vi "init Screen.vi"(8 "error in":errorcluster) -> (0 "error out":errorcluster)   [LabVIEW 2020, in "SimpleDependencyInspector.lvlib"]
uses:
  SimpleDependencyInspector.lvlib
  Image Type--enum.ctl
  Files Selection--cluster.ctl
  File Explorer/File Explorer.lvlib
  <vilib>/Platform/browser.llb/Open URL in Default Browser (string).vi
panel:
  in  "Install Graphviz":bool
  in  "Refresh":bool
  in  "4. Dependency Inspector Working Path":path
  in  "5. Output Image Path":T1
  in  "PPLR":bool caption="Packed Library (*.lvlibp)"
  in  "PPL F":bool caption="Packed Library (*.lvlibp)"
  in  "Virtual Instruments (*.vi) R":bool caption="Virtual Instruments (*.vi)"
  in  "Typedefs(*.ctl) R":bool caption="Typedefs(*.ctl)"
  in  "Class(*.lvclass) R":bool caption="Class(*.lvclass)"
  in  "Libraries(*.lvlib) R":bool caption="Libraries(*.lvlib)"
  in  "Virtual Instruments (*.vi) F":bool caption="Virtual Instruments (*.vi)"
  in  "2. Folder Structure":string[](tree)
  in  "1. LabVIEW Code Folder Container":path
  in  "Typedefs(*.ctl) F":bool caption="Typedefs(*.ctl)"
  in  "Class(*.lvclass) F":bool caption="Class(*.lvclass)"
  in  "Libraries(*.lvlib) F":bool caption="Libraries(*.lvlib)"
  in  "Scan Project":bool caption="8. Find Dependencies from Selection"
  in  "7. Include LV dependencies (vi.lib, usr.lib, etc.)":bool
  # "Instructions:\n1. Choose the folder containing your LabVIEW code.\n2. Select the specific files or folders you want to analyze for dependencies. Use the Shift key to select multiple items.\n3. If you selected folders, specify the LabVIEW file types to include in the analysis.\n4.Specify the Working Path, where the .dot file and dependency image will be saved.\n5. Select the Image type for the dependencies. SVG is the preferred option, LabVIEW cannot handle these images directly. If you choose SVG, the image will be opened in your default browser.\n6.Select the dependency file Types you want to include in your plot.\n7. Decide whether to include all LabVIEW dependencies in the plot. Note that this may result in a large and complex diagram that can be difficult to interpret.\n8.Click the \"Find Dependencies from Selection\" button to begin the analysis."
  # "6. Dependencies to Include in the plot:"
  # "3. Files to Scan for Dependencies in folders:"
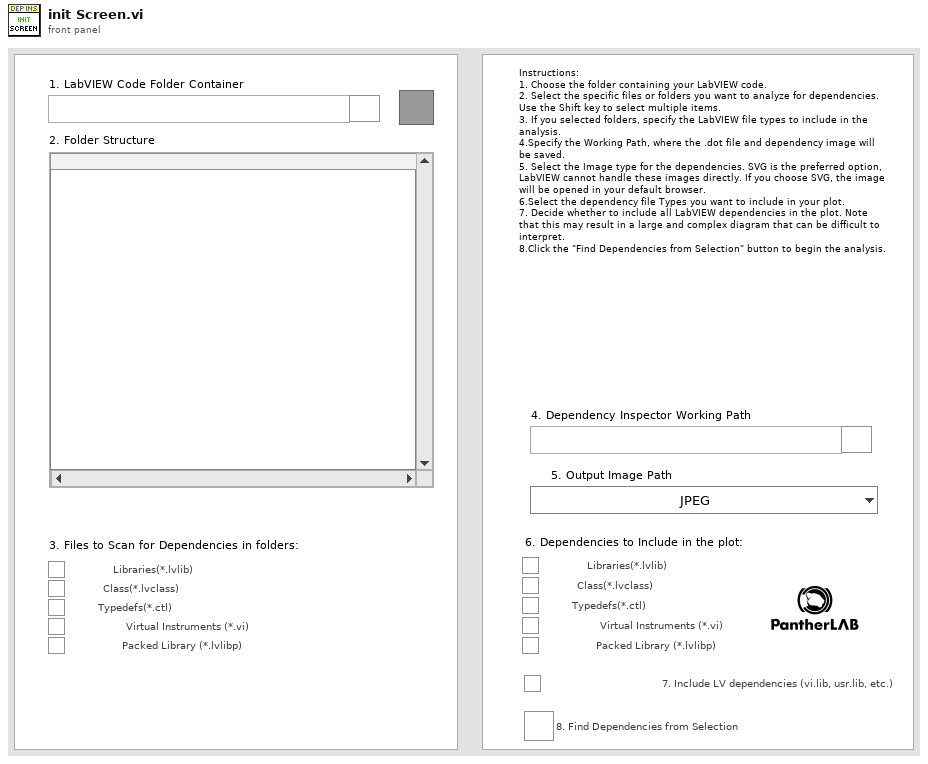
[diagram p1: front panel]
types:
  T1 = typedef "SimpleDependencyInspector.lvlib/Image Type--enum.ctl" = enum16{"JPEG", "PNG", "BMP", "SVG"}
  T2 = typedef "SimpleDependencyInspector.lvlib/Broadcast Events--cluster.ctl" = cluster{"Module Did Init":refnum<user-event>, "Status Updated":refnum<user-event>, "Error Reported":refnum<user-event>, "Module Did Stop":refnum<user-event>, "Update Module Execution Status":refnum<user-event>}
  T3 = typedef "SimpleDependencyInspector.lvlib/Files Selection--cluster.ctl" = cluster{"LVLib":bool, "LVClass":bool, "Typedefs":bool, "vis":bool, "ppl":bool}
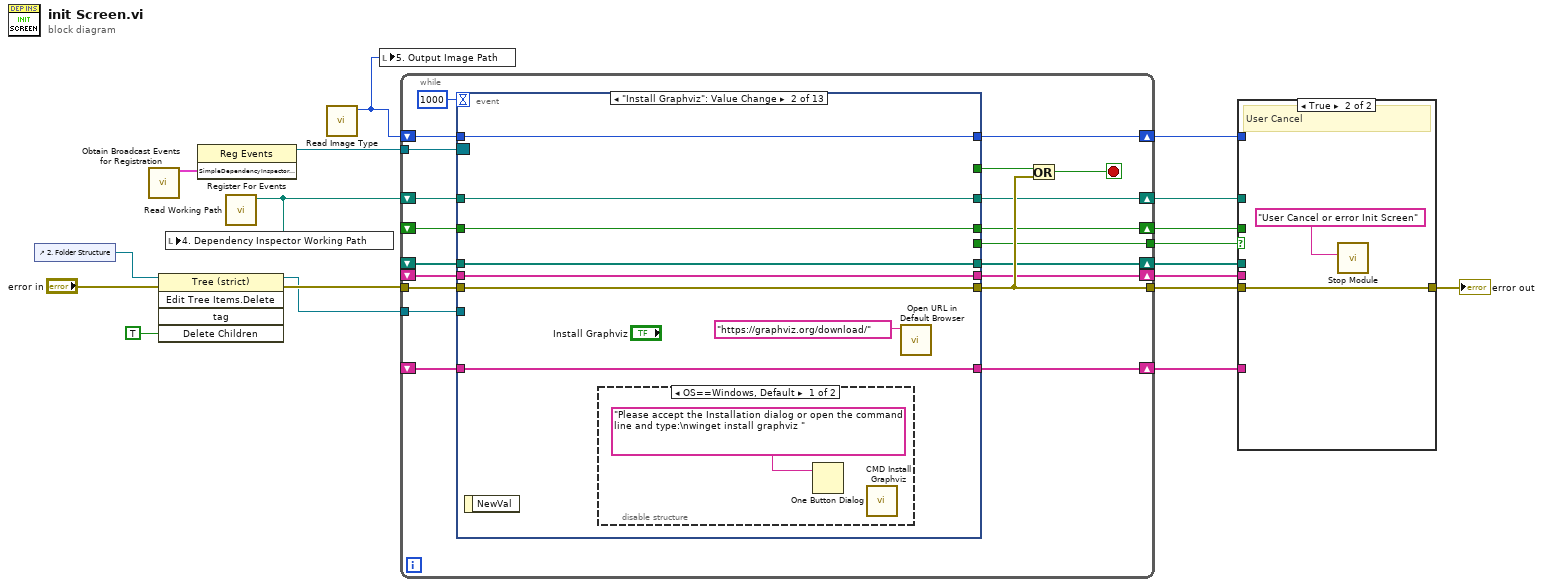
[diagram p0: block diagram]
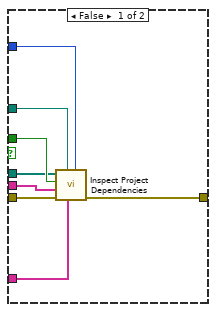
[diagram p2: hidden frame]
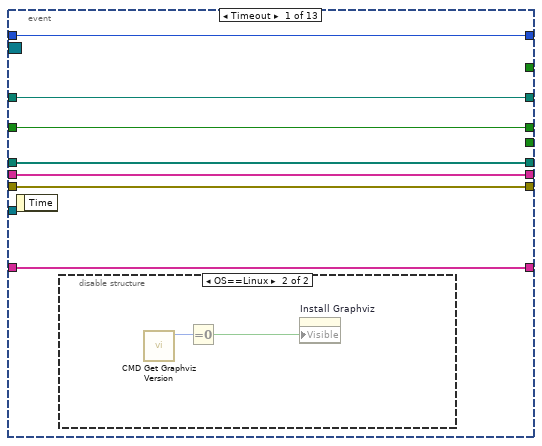
[diagram p3: hidden frame]
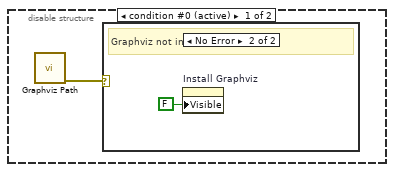
[diagram p4: hidden frame]
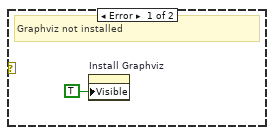
[diagram p5: hidden frame]
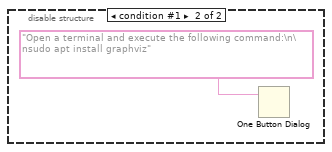
[diagram p6: hidden frame]
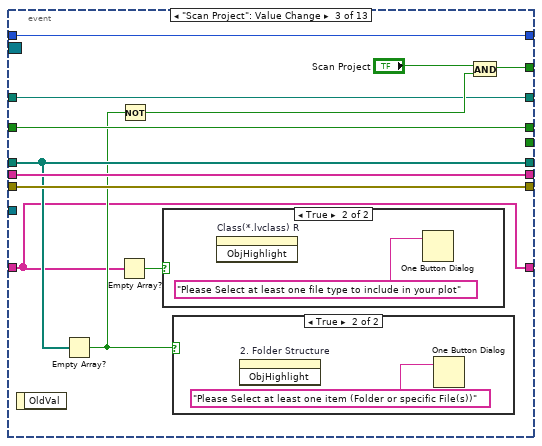
[diagram p7: hidden frame]
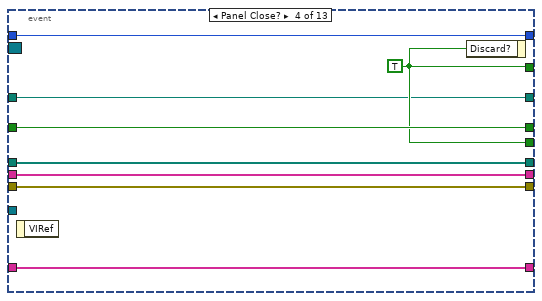
[diagram p10: hidden frame]
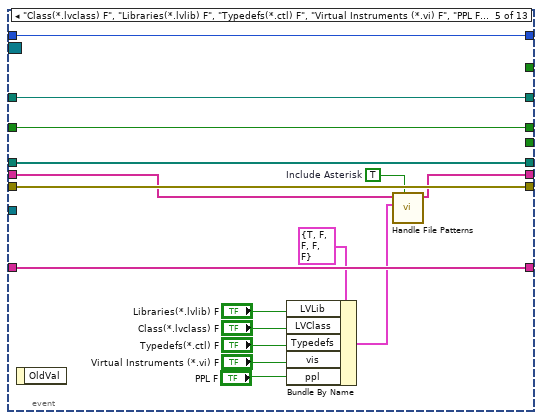
[diagram p11: hidden frame]
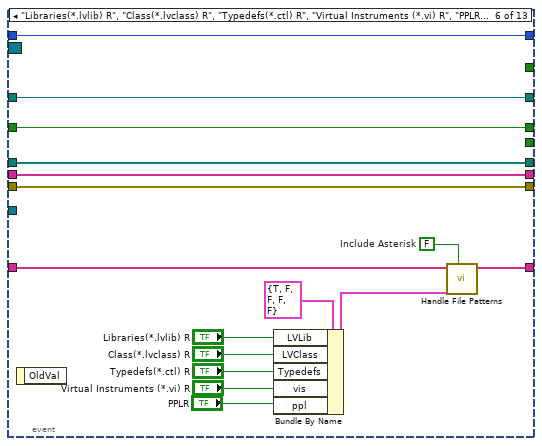
[diagram p12: hidden frame]
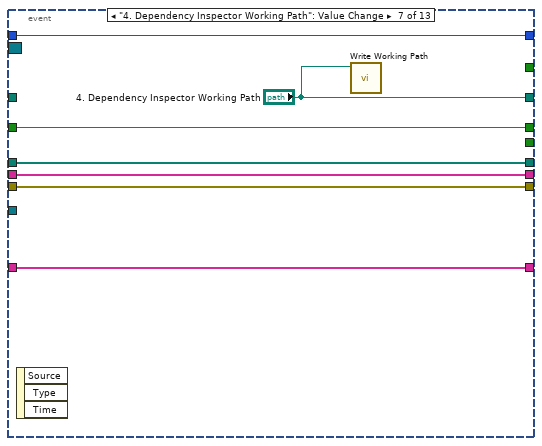
[diagram p13: hidden frame]
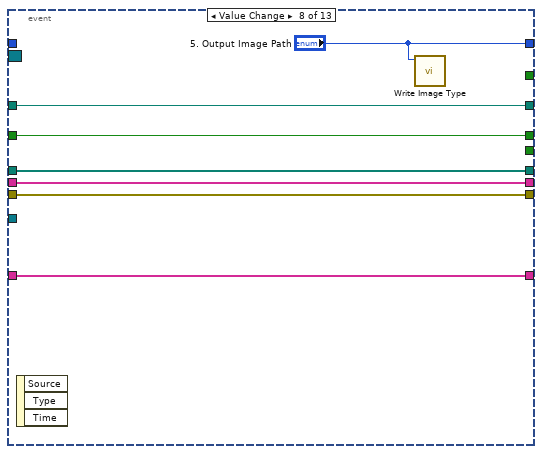
[diagram p14: hidden frame]
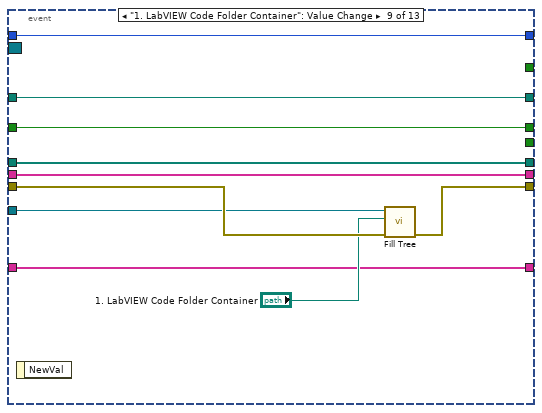
[diagram p15: hidden frame]
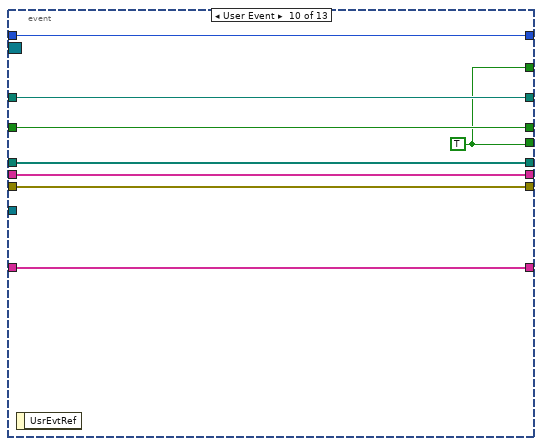
[diagram p16: hidden frame]
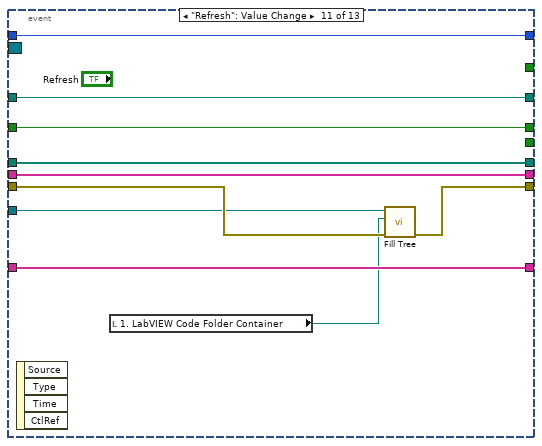
[diagram p17: hidden frame]
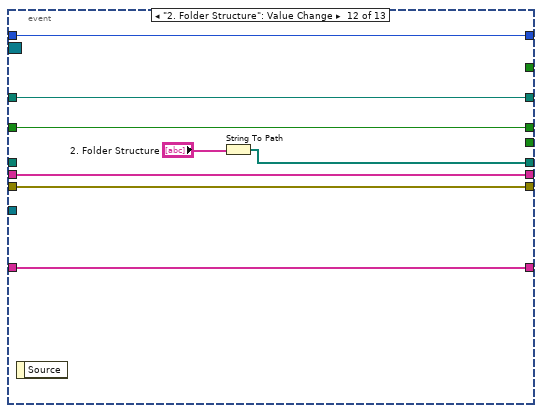
[diagram p18: hidden frame]
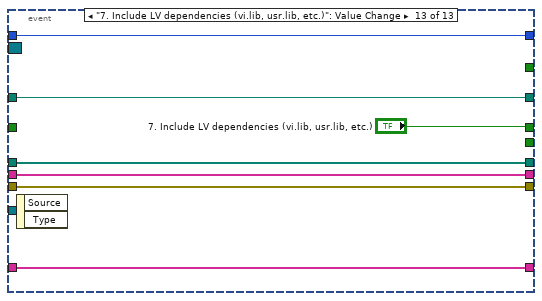
[diagram p19: hidden frame]
diagram:
  n1 = control-ref of="2. Folder Structure"() -> (w11:refnum<vi>)
  n2 = call "Obtain Broadcast Events for Registration.vi"() -> ("SimpleDependencyInspector Broadcast Events"=w5:T2)  [unwired: 9 in, 2 out]
  n3 = invoke class="Tree (strict)" method="Edit Tree Items.Delete"(reference=w11, error in="error in", "Delete Children"=TRUE ("Delete Children?")) -> (reference out=w10:refnum<vi>, error out=w15:errorcluster)  [unwired: 2 in, 3 out]
  n4 = register-events(w5) -> (reference out=w6:refnum<event-registration>)  [unwired: 2 in, 1 out]
  n5 = call "Read Working Path.vi"() -> ("Working Path"=w2:path)  [unwired: 11 in]
  n6 = local write "4. Dependency Inspector Working Path"(w2) -> ()
  n7 = call "Read Image Type.vi"() -> ("Output Image Type"=w1:T1)  [unwired: 11 in]
  n8 = local write "5. Output Image Path"(w1) -> ()
  n9 = while {
    shift-right: [w35] -> w14
    shift-left: _ -> [w34]
    shift-right: [w28] -> w13
    shift-left: _ -> [w33]
    shift-right: [w31] -> w12
    shift-left: _ -> [w32]
    tunnel: w15 -> [w38]
    tunnel: [w37] -> w18
    tunnel: w10 -> [w29]
    tunnel: [w27] -> w9
    shift-right: [w26] -> w8
    shift-left: _ -> [w25]
    tunnel: w6 -> [w24]
    shift-right: [w23] -> w4
    shift-left: w2 -> [w22]
    shift-right: [w21] -> w3
    shift-left: w1 -> [w20]
    stop <- w30 stop-if-true
    n10 = event shown="[1] \"Install Graphviz\": Value Change" {
      selector: w24 -> [_ _ _ _ _ _ _ _ _ _ _ _ _]
      dyn-events: _ -> [_ _ _ _ _ _ _ _ _ _ _ _ _]
      timeout: 1000 -> [_ _ _ _ _ _ _ _ _ _ _ _ _]
      tunnel: w38 -> [w45 w58 w72 w82 w98 w114 w121 w128 w138 w146 w156 w164 w171]
      tunnel: [w45 w58 w72 w82 w98 w114 w121 w128 w137 w146 w155 w164 w171] -> w37
      tunnel: [w42 w57 w66 w79 w94 w112 w120 w127 w132 w145 w151 w160 w169] -> w28
      tunnel: [_ _ w68 w78 _ _ _ _ _ w139 _ _ _] -> w36
      tunnel: [w44 w56 w71 w81 w97 w113 w119 w126 w136 w144 w154 w163 "7. Include LV dependencies (vi.lib, usr.lib, etc.)"] -> w35
      tunnel: w34 -> [w44 w56 w71 w81 w97 w113 w119 w126 w136 w144 w154 w163 _]
      tunnel: w33 -> [w42 w57 w66 w79 w94 w112 w120 w127 w132 w145 w151 _ w169]
      tunnel: w32 -> [w43 w55 w69 w80 w96 w110 w118 w125 w135 w143 w153 w162 w168]
      tunnel: [w43 w55 w69 w80 w95 w110 w118 w125 w135 w143 w153 w162 w168] -> w31
      tunnel: w29 -> [_ _ _ _ _ _ _ _ w134 _ w152 _ _]
      tunnel: [_ _ _ w78 _ _ _ _ _ w139 _ _ _] -> w27
      tunnel: [w41 w54 w64 w77 w92 w109 w117 w124 w131 w142 w150 w159 w167] -> w26
      tunnel: w25 -> [w41 w54 w64 w77 w92 w108 w117 w124 w131 w142 w150 w159 w167]
      tunnel: [w40 w53 w62 w76 w84 w100 "4. Dependency Inspector Working Path" w123 w130 w141 w149 w158 w166] -> w23
      tunnel: w22 -> [w40 w53 w62 w76 w84 w100 _ w123 w130 w141 w149 w158 w166]
      tunnel: [w39 w52 w61 w75 w83 w99 w116 "5. Output Image Path" w129 w140 w148 w157 w165] -> w21
      tunnel: w20 -> [w39 w52 w61 w75 w83 w99 w116 _ w129 w140 w148 w157 w165]
      event Timeout {
        n11 = event-data() -> ()  [unwired: 1 in, 1 out]
        n12 = disable-structure shown="OS==Linux" {
          frame condition #0 (active) {
            n13 = call "Graphviz Path.vi"() -> ("error out"=w46:errorcluster)  [unwired: 10 in, 1 out]
            n14 = case shown="No Error" w46 {
              frame Error {
                # "Graphviz not installed"
                n15 = property on="Install Graphviz" class="Bool"("Visible"=TRUE) -> ()  [unwired: 2 in, 2 out]
              }
              frame No Error {
                # "Graphviz not installed"
                n16 = property on="Install Graphviz" class="Bool"("Visible"=FALSE) -> ()  [unwired: 2 in, 2 out]
              }
            }
          }
          frame condition #1 {
            n17 = call "CMD Get Graphviz Version.vi"() -> ("Mayor Version"=w50:i32)  [unwired: 10 in, 1 out]
            n18 = Equal To 0?(x=w50) -> (x = 0?=w49:bool)
            n19 = property on="Install Graphviz" class="Bool"("Visible"=w49) -> ()  [unwired: 2 in, 2 out]
          }
        }
      }
      event "Install Graphviz": Value Change {
        n20 = event-data() -> ()  [unwired: 1 in, 1 out]
        n21 = disable-structure shown="OS==Windows, Default" {
          frame condition #0 (active) {
            n22 = One Button Dialog(message="Please accept the Installation dialog or open the command line and type:\nwinget install graphviz ") -> ()  [unwired: 1 in, 1 out]
            n23 = call "CMD Install Graphviz.vi"() -> ()  [unwired: 11 in, 1 out]
          }
          frame condition #1 {
            n24 = One Button Dialog(message="Open a terminal and execute the following command:\n\nsudo apt install graphviz") -> ()  [unwired: 1 in, 1 out]
          }
        }
        n25 = call-poly <vilib>:"Open URL in Default Browser.vi"("URL"="https://graphviz.org/download/" ("message")) -> ()  [unwired: 5 in, 2 out]
      }
      event "Scan Project": Value Change {
        n26 = event-data() -> ()  [unwired: 1 in, 1 out]
        n27 = Empty Array?(array=w66) -> (empty?=w65:bool)
        n28 = Empty Array?(array=w64) -> (empty?=w63:bool)
        n29 = Not(x=w65) -> (.not. x?=w67:bool)
        n30 = case shown="True" w63 {
          frame False {
          }
          frame True {
            n31 = invoke on="Class(*.lvclass) R" class="Bool (strict)" method="ObjHighlight"() -> ()  [unwired: 3 in, 3 out]
            n32 = One Button Dialog(message="Please Select at least one file type to include in your plot") -> ()  [unwired: 1 in, 1 out]
          }
        }
        n33 = case shown="True" w65 {
          frame False {
          }
          frame True {
            n34 = invoke on="2. Folder Structure" class="Tree (strict)" method="ObjHighlight"() -> ()  [unwired: 3 in, 3 out]
            n35 = One Button Dialog(message="Please Select at least one item (Folder or specific File(s))") -> ()  [unwired: 1 in, 1 out]
          }
        }
        n36 = And(x="Scan Project", y=w67) -> (x .and. y?=w68:bool)
      }
      event Panel Close? {
        w78 = TRUE ("Discard?")
        n37 = event-data() -> ()  [unwired: 1 in, 1 out]
        n38 = event-data("Discard?"=w78) -> ()  [unwired: 1 in, 1 out]
      }
      event "Class(*.lvclass) F", "Libraries(*.lvlib) F", "Typedefs(*.ctl) F", "Virtual Instruments (*.vi) F", "PPL F": Value Change {
        w93 = TRUE  # Include Asterisk
        n39 = event-data() -> ()  [unwired: 1 in, 1 out]
        n40 = Bundle By Name(cluster=T3 {"LVLib"=TRUE, "LVClass"=FALSE, "Typedefs"=FALSE, "vis"=FALSE, "ppl"=FALSE} ("Files Selection"), "LVLib"="Libraries(*.lvlib) F", "LVClass"="Class(*.lvclass) F", "Typedefs"="Typedefs(*.ctl) F", "vis"="Virtual Instruments (*.vi) F", "ppl"="PPL F") -> (w90:T3)
        n41 = call "Handle File Patterns.vi"("Include Asterisk"=w93, "Files Selection"=w90, "pattern"=w96) -> ("Pattern out"=w95:string[])  [unwired: 8 in]
      }
      event "Libraries(*.lvlib) R", "Class(*.lvclass) R", "Typedefs(*.ctl) R", "Virtual Instruments (*.vi) R", "PPLR": Value Change {
        w111 = FALSE  # Include Asterisk
        n42 = event-data() -> ()  [unwired: 1 in, 1 out]
        n43 = Bundle By Name(cluster=T3 {"LVLib"=TRUE, "LVClass"=FALSE, "Typedefs"=FALSE, "vis"=FALSE, "ppl"=FALSE} ("Files Selection"), "LVLib"="Libraries(*.lvlib) R", "LVClass"="Class(*.lvclass) R", "Typedefs"="Typedefs(*.ctl) R", "vis"="Virtual Instruments (*.vi) R", "ppl"="PPLR") -> (w106:T3)
        n44 = call "Handle File Patterns.vi"("Include Asterisk"=w111, "Files Selection"=w106, "pattern"=w108) -> ("Pattern out"=w109:string[])  [unwired: 8 in]
      }
      event "4. Dependency Inspector Working Path": Value Change {
        n45 = event-data() -> ()  [unwired: 1 in, 3 out]
        n46 = call "Write Working Path.vi"("Working Path"="4. Dependency Inspector Working Path") -> ()  [unwired: 11 in]
      }
      event Value Change {
        n47 = event-data() -> ()  [unwired: 1 in, 3 out]
        n48 = call "Write Image Type.vi"("Output Image Type"="5. Output Image Path") -> ()  [unwired: 11 in]
      }
      event "1. LabVIEW Code Folder Container": Value Change {
        n49 = event-data() -> ()  [unwired: 1 in, 1 out]
        n50 = call "Fill Tree.vi"("error in"=w138, "Folder Path"="1. LabVIEW Code Folder Container", "TreeControl in"=w134) -> ("error out"=w137:errorcluster)  [unwired: 8 in]
      }
      event User Event {
        w139 = TRUE ("Discard?")
        n51 = event-data() -> ()  [unwired: 1 in, 1 out]
      }
      event "Refresh": Value Change {
        n52 = event-data() -> ()  [unwired: 1 in, 4 out]
        n53 = local read "1. LabVIEW Code Folder Container"() -> (w147:path)
        n54 = call "Fill Tree.vi"("error in"=w156, "Folder Path"=w147, "TreeControl in"=w152) -> ("error out"=w155:errorcluster)  [unwired: 8 in]
      }
      event "2. Folder Structure": Value Change {
        n55 = event-data() -> ()  [unwired: 1 in, 1 out]
        n56 = String To Path(string="2. Folder Structure") -> (path=w160:path[])
      }
      event "7. Include LV dependencies (vi.lib, usr.lib, etc.)": Value Change {
        n57 = event-data() -> ()  [unwired: 1 in, 2 out]
      }
    }
    n58 = Or(x=w36, y=w37) -> (x .or. y?=w30:bool)
  }
  n59 = case shown="True" w9 {
    tunnel: [w178 w181] -> w17
    tunnel: w14 -> [w177 _]
    tunnel: w13 -> [w175 _]
    tunnel: w12 -> [w176 _]
    tunnel: w18 -> [w179 w181]
    tunnel: w8 -> [w174 _]
    tunnel: w4 -> [w173 _]
    tunnel: w3 -> [w172 _]
    frame False {
      n60 = call "Inspect Project Dependencies.vi"("Img Type"=w172, "pattern To include in Plot"=w174, "Working Path"=w173, "error in"=w179, "pattern"=w176, "Include vi.lib"=w177, "Path(s) Selection"=w175) -> ("error out"=w178:errorcluster)  [unwired: 4 in]
    }
    frame True {
      # "User Cancel"
      n61 = call "Stop Module.vi"("Origin"="User Cancel or error Init Screen") -> ()  [unwired: 10 in, 1 out]
    }
  }
  "error out" <- w17
